vi "cryocon ramp to temperature.vi"(8 "error in (no error)":errorcluster, 9 "stability (K)":dbl=0.01, 10 "target temperature (K)":dbl, 11 "VISA resource name":refnum<visa-resource-name>="GPIB1::12::INSTR") -> (0 "error out":errorcluster, 3 "VISA resource name":refnum<visa-resource-name>)   [LabVIEW 2013]
uses:
  config.vi
panel:
  # "Sets the target temperature of the sample."
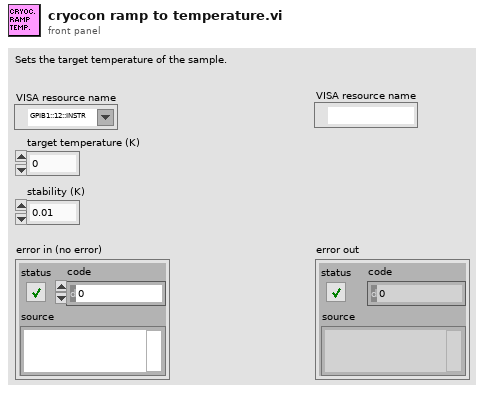
[diagram p1: front panel]
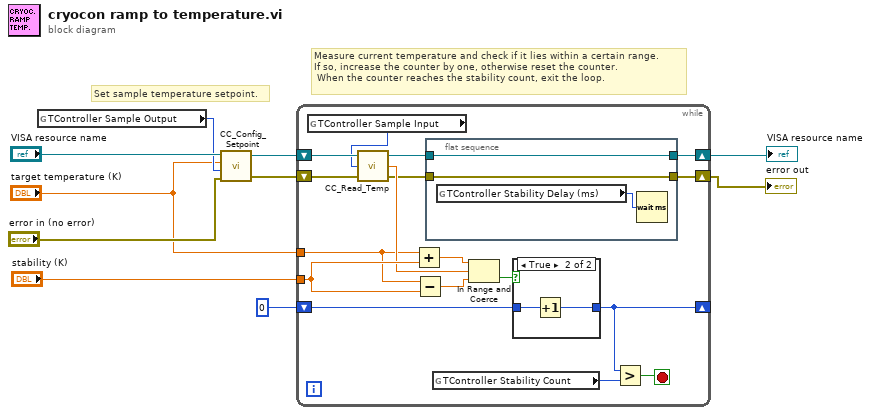
[diagram p0: block diagram]
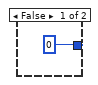
[diagram p2: hidden frame]
diagram:
  # "Measure current temperature and check if it lies within a certain range.\nIf so, increase the counter by one, otherwise reset the counter.\n When the counter reaches the stability count, exit the loop."
  # "Set sample temperature setpoint."
  n1 = global read "config.vi" "TController Sample Output"() -> (w4:u8)
  n2 = call <userlib>:"CC_Config_Setpoint.vi"("error in (no error)"="error in (no error)", "Output"=w4, "Set Point"="target temperature (K)", "VISA In"="VISA resource name") -> ("error out"=w6:errorcluster, "VISA Out"=w7:refnum<visa-resource-name>)  [unwired: 1 out]
  n3 = while {
    shift-right: [w12] -> _
    shift-left: 0 ("target temperature (K)") -> [w13]
    tunnel: "stability (K)" -> [w24]
    shift-right: [w18] -> w3
    shift-left: w7 -> [w27]
    shift-right: [w16] -> w2
    shift-left: w6 -> [w26]
    tunnel: "target temperature (K)" -> [w11]
    stop <- w20 stop-if-true
    n4 = global read "config.vi" "TController Sample Input"() -> (w15:u8)
    n5 = call <userlib>:"CC_Read_Temp.vi"("error in (no error)"=w26, "Input"=w15, "VISA In"=w27) -> ("error out"=w17:errorcluster, "Temperature"=w23:dbl, "VISA Out"=w19:refnum<visa-resource-name>)
    n6 = Add(x=w11, y=w24) -> (x+y=w25:dbl)
    n7 = Subtract(x=w11, y=w24) -> (x-y=w22:dbl)
    n8 = flat-sequence {
      tunnel: w19 -> [w30]
      tunnel: [w30] -> w18
      tunnel: w17 -> [w29]
      tunnel: [w29] -> w16
      frame #0 {
        n9 = global read "config.vi" "TController Stability Delay (ms)"() -> (w28:i32)
        n10 = Wait (ms)(milliseconds to wait=w28) -> ()  [unwired: 1 out]
      }
    }
    n11 = global read "config.vi" "TController Stability Count"() -> (w14:i32)
    n12 = In Range and Coerce(upper limit=w25, x=w23, lower limit=w22) -> (In Range?=w21:bool)  [unwired: 1 out]
    n13 = case shown="True" w21 {
      tunnel: w13 -> [_ w33]
      tunnel: [0 ("target temperature (K)") w32] -> w12
      frame False {
      }
      frame True {
        n14 = Increment(x=w33) -> (x+1=w32:i32)
      }
    }
    n15 = Greater?(x=w12, y=w14) -> (0:w20:bool)
  }
  "VISA resource name" <- w3
  "error out" <- w2
